vi "FTW-Collection-JSON-Deserialize.vi"(0 "Collection":refnum<class "FTW-Collection.lvclass">, 5 "Serialized Collection":string, 11 "error in":errorcluster) -> (4 "Collection out":refnum<class "FTW-Collection.lvclass">, 6 "Valid Structure":bool, 15 "error out":errorcluster)   [LabVIEW 2013, in "FTW-Collection.lvclass"]
uses:
  FTW-Collection.lvclass
panel:
  # "Inputs"
  # "Outputs"
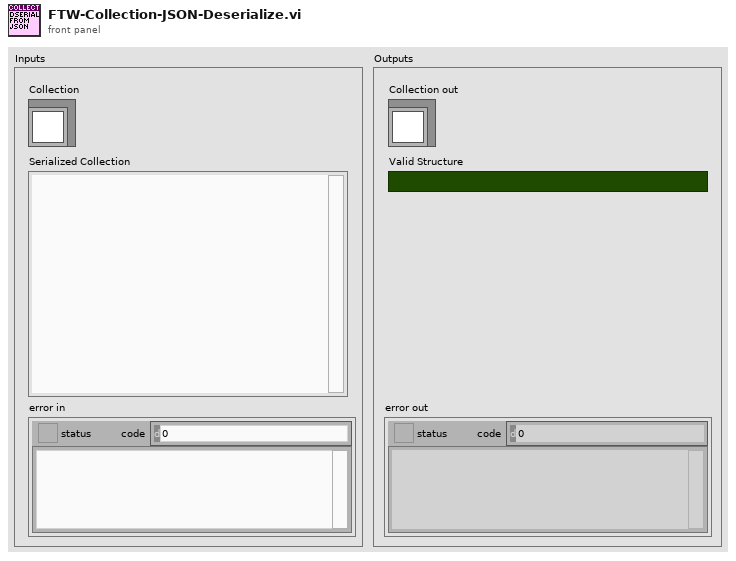
[diagram p1: front panel]
types:
  T1 = typedef "FTW-Collection-KeyValuePair.ctl" = cluster{"Key":string, "Value":string}
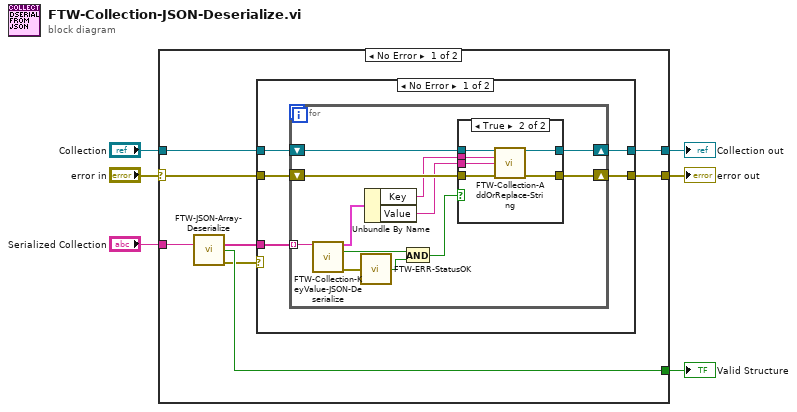
[diagram p0: block diagram]
diagram:
  n1 = case shown="No Error" "error in" {
    selector: "error in" -> [w13 w43]
    tunnel: [w12 w43] -> w6
    tunnel: "Collection" -> [w14 w42]
    tunnel: [w11 w42] -> w3
    tunnel: "Serialized Collection" -> [w10 _]
    tunnel: [w9 _] -> w1
    frame No Error {
      n2 = call "FTW-JSON-Array-Deserialize.vi"("Array of JSON Objects"=w10) -> ("JSON Elements"=w7:string[], "Valid Structure"=w9:bool, "error out"=w8:errorcluster)  [unwired: 12 in]
      n3 = case shown="No Error" w8 {
        tunnel: w14 -> [w19 w41]
        tunnel: w13 -> [w18 w40]
        tunnel: [w17 w40] -> w12
        tunnel: [w16 w41] -> w11
        tunnel: w7 -> [w15 _]
        frame No Error {
          n4 = for {
            tunnel: w15 -> [w25] mode=indexing
            shift-right: [w29] -> w16
            shift-left: w19 -> [w31]
            shift-right: [w26] -> w17
            shift-left: w18 -> [w27]
            n5 = call "FTW-Collection-KeyValue-JSON-Deserialize.vi"("Serialized Key-Value Pair"=w25) -> ("Key-Value Pair"=w22:T1, "Valid Structure"=w24:bool, "error out"=w23:errorcluster)  [unwired: 12 in]
            n6 = call "FTW-ERR-StatusOK.vi"("error to check"=w23) -> ("Status OK?"=w30:bool)
            n7 = Unbundle By Name(w22) -> ("Key"=w21:string, "Value"=w20:string)
            n8 = And(x=w24, y=w30) -> (x .and. y?=w28:bool)
            n9 = case shown="True" w28 {
              tunnel: w31 -> [w33 w39]
              tunnel: w21 -> [_ w38]
              tunnel: w20 -> [_ w37]
              tunnel: [w33 w36] -> w29
              tunnel: w27 -> [w32 w35]
              tunnel: [w32 w34] -> w26
              frame False {
              }
              frame True {
                n10 = call "FTW-Collection-AddOrReplace-String.vi"("Collection"=w39, "Key"=w38, "Value"=w37, "error in"=w35) -> ("Collection out"=w36:refnum<class "FTW-Collection.lvclass">, "error out"=w34:errorcluster)  [unwired: 9 in, 1 out]
              }
            }
          }
        }
        frame Error {
        }
      }
    }
    frame Error {
    }
  }
  "error out" <- w6
  "Collection out" <- w3
  "Valid Structure" <- w1
